vi "Calculate CO2 (2).vi"(7 "Use Channel":u8=1 min=1 max=4, 9 "BreathDuration":dbl, 10 "Daq Needed":T1 {"Current Settings"."Pump" items=["Pump 0", "Pump 1", "Pump 2", "Pump 3", "Pump 4", "Pump 5"]; "Current Settings"."Chart X axis Timescale" min=20 max=180 step=1; "Current Settings"."RunTime Mode Settings"."Exp. Gas Tank" items=["0.07", "0.031", "0.877", "1.863", "3.881", "5.790", "7.688", "6.000"]; "Current Settings"."RunTime Mode Settings"."Insp. Gas Tank" items=["0.07", "0.031", "0.877", "1.863", "3.881", "5.790", "7.688", "6.000"]; "Current Settings"."RunTime Mode Settings"."I:E Ratio" max=30 scale=0.0..7.0; "Current Settings"."RunTime Mode Settings"."Resp Rate Brpm" min=0 max=30 format="%.2f"; "Current Settings"."TE#2 Configuration"."Serial Port"."XOFF Char" format="%.0x"; "Current Settings"."TE#2 Configuration"."Serial Port"."XON Char" format="%.0x"; "Current Settings"."TE#2 Configuration"."Serial Port"."flow control" items=["None"=0, "XON/XOFF"=1, "RTS/CTS"=2, "DTR/DSR"=4]; "Current Settings"."TE#2 Configuration"."Serial Port"."stop bits" items=["1.0"=10, "1.5"=15, "2.0"=20]; "Current Settings"."TE#2 Configuration"."Serial Port"."data bits" min=5 max=8 step=1; "Current Settings"."TE#2 Configuration"."Serial Port"."baud rate" items=["75"=75, "110"=110, "134"=134, "150"=150, "300"=300, "600"=600, "1200"=1200, "1800"=1800, "2400"=2400, "4800"=4800, "7200"=7200, "9600"=9600, "14400"=14400, "19200"=19200, "28800"=28800, "38400"=38400, "56000"=56000, "57600"=57600, "115200"=115200, "128000"=128000, "230400"=230400]; "Current Settings"."TE#2 Configuration"."Serial Port"."termination char" format="%.0x"; "Current Settings"."TE#1 Configuration"."Serial Port"."XOFF Char" format="%.0x"; "Current Settings"."TE#1 Configuration"."Serial Port"."XON Char" format="%.0x"; "Current Settings"."TE#1 Configuration"."Serial Port"."flow control" items=["None"=0, "XON/XOFF"=1, "RTS/CTS"=2, "DTR/DSR"=4]; "Current Settings"."TE#1 Configuration"."Serial Port"."stop bits" items=["1.0"=10, "1.5"=15, "2.0"=20]; "Current Settings"."TE#1 Configuration"."Serial Port"."data bits" min=5 max=8 step=1; "Current Settings"."TE#1 Configuration"."Serial Port"."baud rate" items=["75"=75, "110"=110, "134"=134, "150"=150, "300"=300, "600"=600, "1200"=1200, "1800"=1800, "2400"=2400, "4800"=4800, "7200"=7200, "9600"=9600, "14400"=14400, "19200"=19200, "28800"=28800, "38400"=38400, "56000"=56000, "57600"=57600, "115200"=115200, "128000"=128000, "230400"=230400]; "Current Settings"."TE#1 Configuration"."Serial Port"."termination char" format="%.0x"; "Current Settings"."Capnometer Configuration"."Device" items=["None", "TidalWave", "LoFlow / Canary", "Capnogard"]; "Current Settings"."Capnometer Configuration"."Serial Port"."XOFF Char" format="%.0x"; "Current Settings"."Capnometer Configuration"."Serial Port"."XON Char" format="%.0x"; "Current Settings"."Capnometer Configuration"."Serial Port"."flow control" items=["None"=0, "XON/XOFF"=1, "RTS/CTS"=2, "DTR/DSR"=4]; "Current Settings"."Capnometer Configuration"."Serial Port"."stop bits" items=["1.0"=10, "1.5"=15, "2.0"=20]; "Current Settings"."Capnometer Configuration"."Serial Port"."data bits" min=5 max=8 step=1; "Current Settings"."Capnometer Configuration"."Serial Port"."baud rate" items=["75"=75, "110"=110, "134"=134, "150"=150, "300"=300, "600"=600, "1200"=1200, "1800"=1800, "2400"=2400, "4800"=4800, "7200"=7200, "9600"=9600, "14400"=14400, "19200"=19200, "28800"=28800, "38400"=38400, "56000"=56000, "57600"=57600, "115200"=115200, "128000"=128000, "230400"=230400]; "Current Settings"."Capnometer Configuration"."Serial Port"."termination char" format="%.0x"; "Current Settings"."DAQx Settings"."Analog Output Settings (Volts)" format="%#.3g"; "Current Settings"."DAQx Settings"."Duty Cycle" min=10.0 max=90.0 format="%.1g"; "Current Settings"."DAQx Settings"."Frequency" min=20.0 max=200.0; "Current Settings"."DataLogging Settings"."Data File Duration (Minutes)" min=2 max=200 format="%#.2g"; "Current Settings"."Calibration Settings"."Tolerance #2" min=2 max=4096; "Current Settings"."Calibration Settings"."Cal. Average" min=2 max=4096; "Current Settings"."Test Settings"."Test Sensor ID" items=["(select)", "RB", "YC", "", "Other"]}, 11 "Processed Variables":T9 {"Chamber Temperature" format="%.2f"; "Ambient Temperature" format="%.2f"; "Bath Temperature" format="%.2f"; "Det. Temperature" format="%.2f"; "Detector Chl 4" format="%.2g"; "Detector Chl 3" format="%.2g"; "Ref CO2" format="%.2g"; "Detector Chl 2" format="%.2g"; "Film Temperature" format="%.2f"; "Humidity" format="%.2f"; "Detector Chl 1" format="%.2g"}) -> (1 "RR Out":dbl, 2 "Raws":sgl[](array[numeric]), 3 "ETCO2 Out":dbl, 4 "New Breath Found":bool)   [LabVIEW 2015]
uses:
  Controls/Processed Variables.ctl
  Controls/DAQ Needed.ctl
  Controls/AirPump Controls.ctl
  Controls/IE Ratio knob.ctl
  Controls/UI Settings.ctl
  Controls/Aux CO2 Control.ctl
  Controls/Serial Visa Control.ctl
  Controls/Aux CO2 Selector.ctl
  Controls/Aux TE Control.ctl
  Controls/Queues And Others.ctl
  Miscellaneous/Globals.vi
panel:
  in  "Use New V2C":bool=TRUE
  out "PeakCO2Out":dbl
  # "Note: Setting Brpm to zero will\ndisable Insp / Exp digital output."
  # "mmHg"
  # "pts"
  # "tolerance"
  # "AN5 (Temp 1)"
  # "AN6 (Temp 2)"
  # "AN7 (Temp 3)"
  # "AN8 (T FET)"
  # "AN0 (T POT)"
  # "Tref (Set Pt))"
  # "(Spare)"
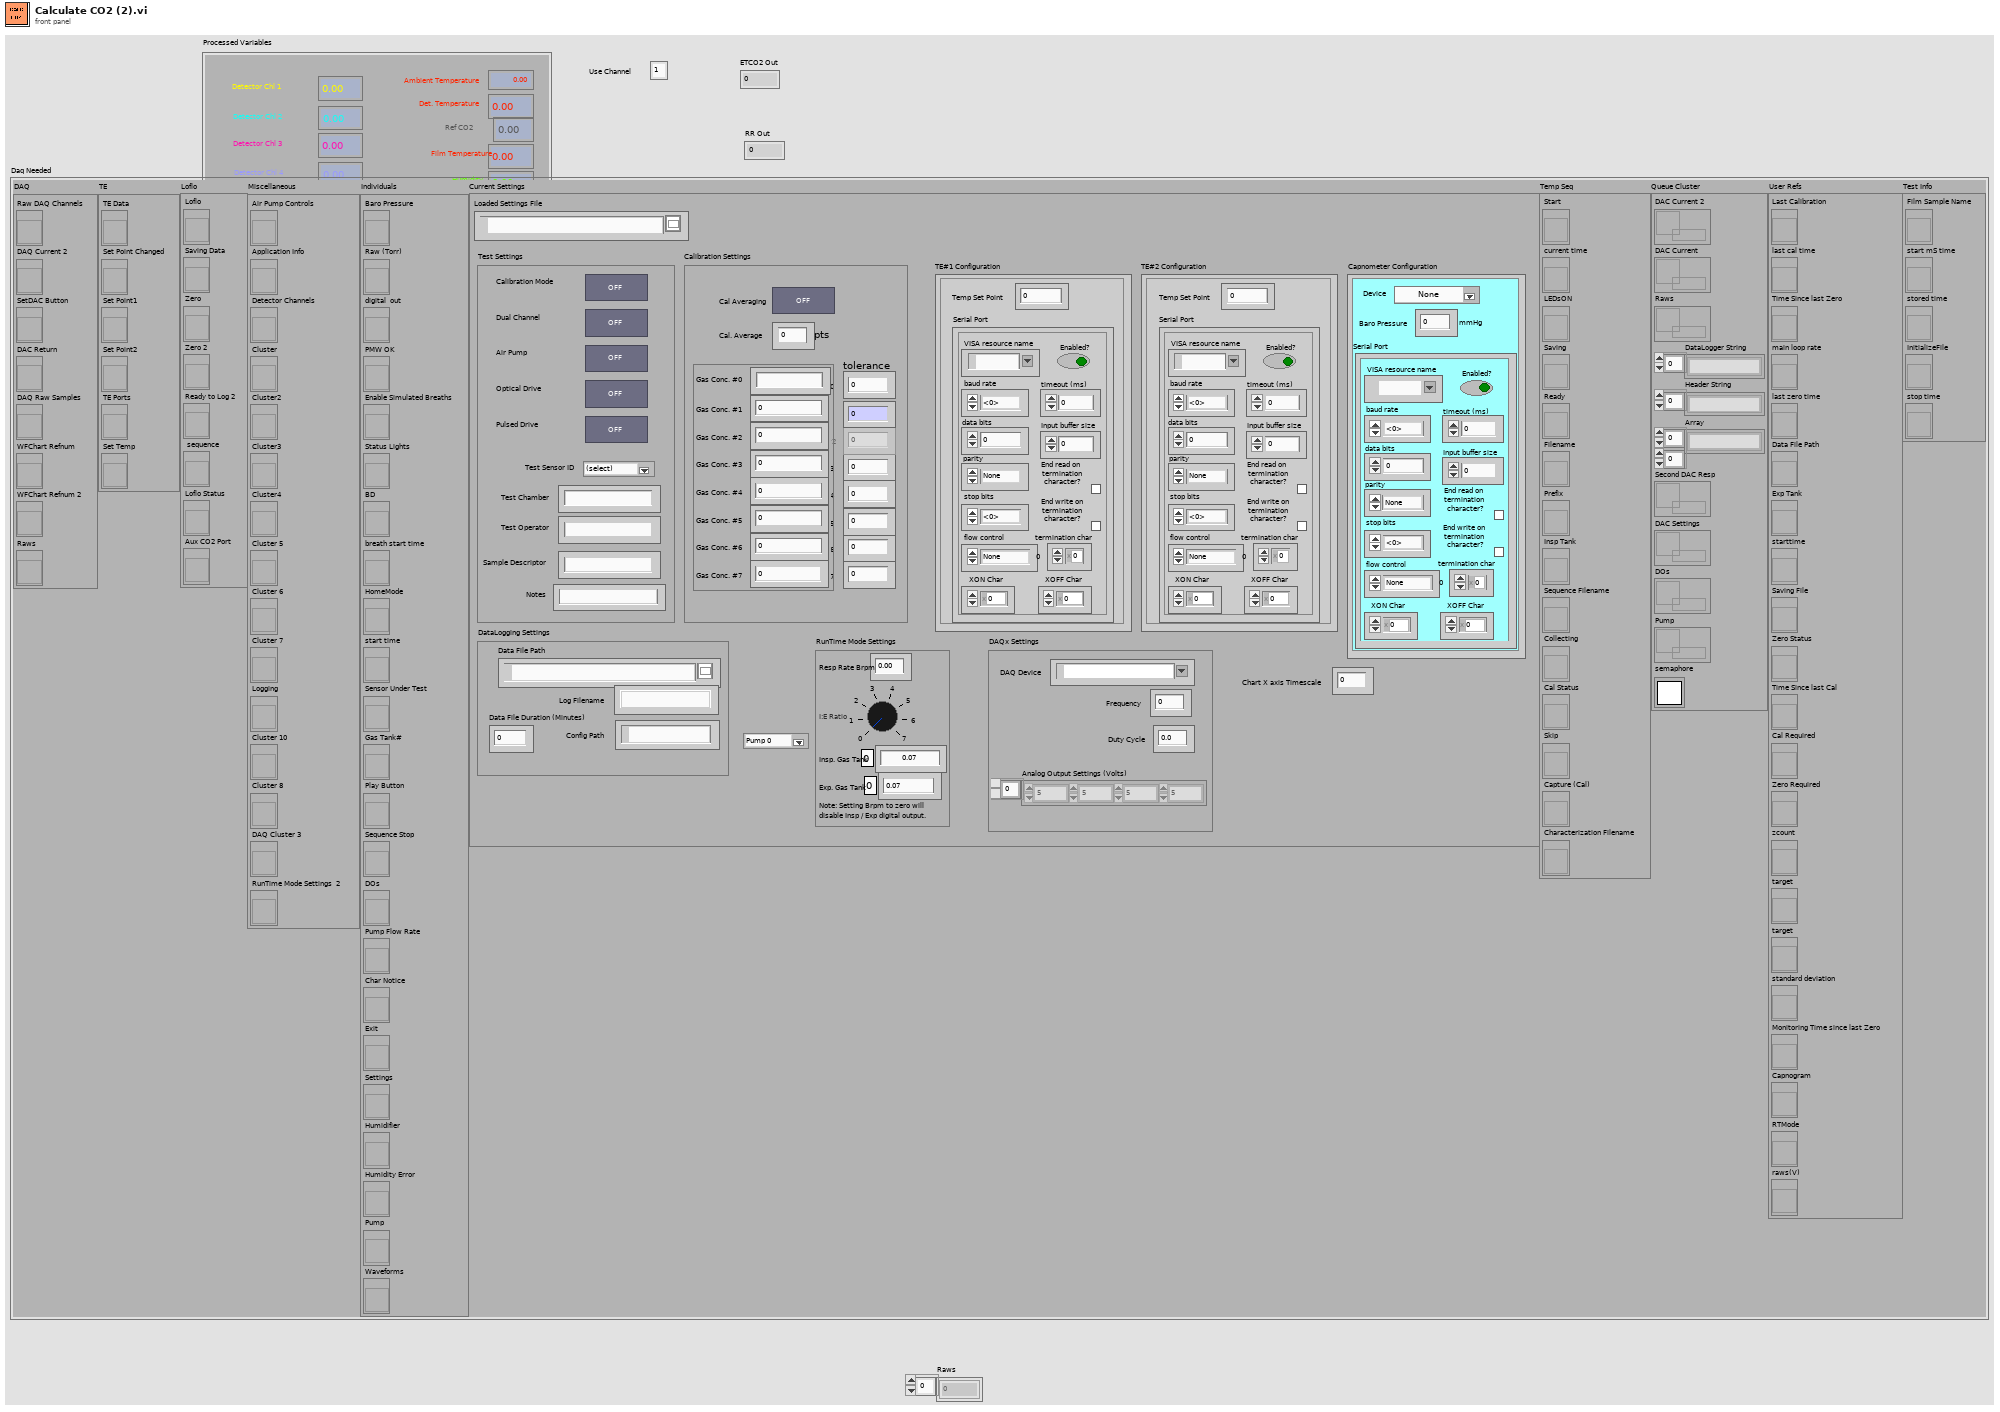
[diagram p1: front panel]
types:
  T1 = typedef "DAQ Needed.ctl" = cluster{"DAQ":cluster{"Raw DAQ Channels":refnum<vi>, "DAQ Current 2":refnum<vi>, "SetDAC Button":refnum<vi>, "DAC Return":refnum<vi>, "DAQ Raw Samples":refnum<vi>, "WFChart Refnum":refnum<vi>, "WFChart Refnum 2":refnum<vi>, "Raws":refnum<vi>}, "TE":cluster{"TE Data":refnum<vi>, "Set Point Changed":refnum<vi>, "Set Point1":refnum<vi>, "Set Point2":refnum<vi>, "TE Ports":refnum<vi>, "Set Temp":refnum<vi>}, "Loflo":cluster{"Loflo":refnum<vi>, "Saving Data":refnum<vi>, "Zero":refnum<vi>, "Zero 2":refnum<vi>, "Ready to Log 2":refnum<vi>, " sequence":refnum<vi>, "Loflo Status ":refnum<vi>, "Aux CO2 Port":refnum<vi>}, "Miscellaneous":cluster{"Air Pump Controls":refnum<vi>, "Application Info":refnum<vi>, "Detector Channels ":refnum<vi>, "Cluster":refnum<vi>, "Cluster2":refnum<vi>, "Cluster3":refnum<vi>, "Cluster4":refnum<vi>, "Cluster 5":refnum<vi>, "Cluster 6":refnum<vi>, "Cluster 7":refnum<vi>, "Logging":refnum<vi>, "Cluster 10":refnum<vi>, "Cluster 8":refnum<vi>, "DAQ Cluster 3":refnum<vi>, "RunTime Mode Settings  2":refnum<vi>}, "Individuals":cluster{"Baro Pressure":refnum<vi>, "Raw (Torr)":refnum<vi>, "digital  out":refnum<vi>, "PMW OK":refnum<vi>, "Enable Simulated Breaths":refnum<vi>, "Status Lights":refnum<vi>, "BD":refnum<vi>, "breath start time":refnum<vi>, "HomeMode":refnum<vi>, "start time":refnum<vi>, "Sensor Under Test":refnum<vi>, "Gas Tank#":refnum<vi>, "Play Button":refnum<vi>, "Sequence Stop":refnum<vi>, "DOs":refnum<vi>, "Pump Flow Rate":refnum<vi>, "Char Notice":refnum<vi>, "Exit":refnum<vi>, "Settings":refnum<vi>, "Humidifier":refnum<vi>, "Humidity Error":refnum<vi>, "Pump":refnum<vi>, "Waveforms":refnum<vi>}, "Current Settings":T2, "Temp Seq":cluster{"Start":refnum<vi>, "current time":refnum<vi>, "LEDsON":refnum<vi>, "Saving":refnum<vi>, "Ready":refnum<vi>, "Filename":refnum<vi>, "Prefix":refnum<vi>, "Insp Tank":refnum<vi>, "Sequence Filename":refnum<vi>, "Collecting":refnum<vi>, "Cal Status":refnum<vi>, "Skip":refnum<vi>, "Capture (Cal)":refnum<vi>, "Characterization Filename":refnum<vi>}, "Queue Cluster":T7, "User Refs":cluster{"Last Calibration":refnum<vi>, "last cal time":refnum<vi>, "Time Since last Zero":refnum<vi>, "main loop rate":refnum<vi>, "last zero time":refnum<vi>, "Data File Path":refnum<vi>, "Exp Tank":refnum<vi>, "starttime":refnum<vi>, "Saving File":refnum<vi>, "Zero Status":refnum<vi>, "Time Since last Cal":refnum<vi>, "Cal Required":refnum<vi>, "Zero Required":refnum<vi>, "zcount":refnum<vi>, "target":refnum<vi>, "target":refnum<vi>, "standard deviation":refnum<vi>, "Monitoring Time since last Zero":refnum<vi>, "Capnogram":refnum<vi>, "RTMode":refnum<vi>, "raws(V)":refnum<vi>}, "Test Info":cluster{"Film Sample Name":refnum<vi>, "start mS time":refnum<vi>, "stored time":refnum<vi>, "InitializeFile":refnum<vi>, "stop time":refnum<vi>}}
  T2 = typedef "UI Settings.ctl" = cluster{"Loaded Settings File":path, "Test Settings":cluster{"Dual Channel":bool, "Air Pump":bool, "Optical Drive":bool, "Pulsed Drive":bool, "Calibration Mode":bool, "Test Sensor ID":u16, "Test Chamber":string, "Test Operator":string, "Sample Descriptor":string, "Notes":string}, "Calibration Settings":cluster{"Cal. Average":u16, "Cal Averaging":bool, "Tolerance #0":sgl, "Tolerance #7":sgl, "Tolerance #6":sgl, "Tolerance #5":sgl, "Tolerance #4":sgl, "Tolerance #3":sgl, "Tolerance #2":sgl, "Tolerance #1":sgl, "Gas Tank Settings":cluster{"Gas Conc. #0":string, "Gas Conc. #1":sgl, "Gas Conc. #2":sgl, "Gas Conc. #3":sgl, "Gas Conc. #4":sgl, "Gas Conc. #5":sgl, "Gas Conc. #6":sgl, "Gas Conc. #7":sgl}}, "DataLogging Settings":cluster{"Data File Path":path, "Data File Duration (Minutes)":sgl, "Log Filename":string, "Config Path":path}, "DAQx Settings":cluster{"DAQ Device":tag, "Frequency":dbl, "Duty Cycle":dbl, "Analog Output Settings (Volts)":sgl[]}, "Capnometer Configuration":T3, "TE#1 Configuration":T6, "TE#2 Configuration":T6, "RunTime Mode Settings ":cluster{"Resp Rate Brpm ":sgl, "I:E Ratio":u8, "Insp. Gas Tank":u16, "Exp. Gas Tank":u16}, "Chart X axis Timescale":u16, "Pump":u16}
  T3 = typedef "Aux CO2 Control.ctl" = cluster{"Serial Port":T4, "Baro Pressure":u32, "Device":T5}
  T4 = typedef "Serial Visa Control.ctl" = cluster{"termination char":u8, "End read on termination character?":bool, "Enabled?":bool, "VISA resource name":refnum<visa-resource-name>, "baud rate":u32, "data bits":u16, "parity":enum16{"None", "Odd", "Even", "Mark", "Space"}, "stop bits":u16, "flow control":u16, "timeout (ms)":u32, "Input buffer size":u32, "End write on termination character?":bool, "XON Char":u8, "XOFF Char":u8}
  T5 = typedef "Aux CO2 Selector.ctl" = u16
  T6 = typedef "Aux TE Control.ctl" = cluster{"Temp Set Point":sgl, "Serial Port":T4}
  T7 = typedef "Queues And Others.ctl" = cluster{"DAC Current 2":refnum<queue>, "DAC Current":refnum<queue>, "Raws":refnum<queue>, "DataLogger String":string[], "Header String":string[], "Array":string[][], "Second DAC Resp":refnum<queue>, "DAC Settings":refnum<queue>, "DOs":refnum<queue>, "Pump":refnum<queue>, "semaphore":T8}
  T8 = typedef "Semaphore RefNum" = refnum<k1>
  T9 = typedef "Processed Variables.ctl" = cluster{"Detector Chl 1":sgl, "Humidity":dbl, "Film Temperature":dbl, "Detector Chl 2":sgl, "Ref CO2":sgl, "Detector Chl 3":sgl, "Detector Chl 4":sgl, "Det. Temperature":dbl, "Bath Temperature":dbl, "Ambient Temperature":dbl, "rt Baro Pressure":u16, "Chamber Temperature":dbl}
  T10 = typedef "Calibration Coefficients.ctl" = cluster{"CalFile Used":path, "TYPE":string, "DATE":string, "Humidity":sgl, "Chamber Temp":dbl, "CO2_calgas":dbl, "V_(RA,5mA)":dbl, "V_(RA,15mA)":dbl, "mI":dbl, "V_0d_ImA (actual)":dbl, "V_6d_ImA (actual)":dbl, "I_span":dbl, "DAC":u16, "A":dbl, "B":dbl, "C":dbl, "D":dbl, "V6d":dbl, "A'":dbl, "B'":dbl, "C'":dbl, "D'":dbl, "V0d":dbl, "CalDate":string, "CalTime":string, "duration":dbl, "Detector Channel":string, "a2":dbl, "a3":dbl, "a4":dbl, "a5":dbl, "b2":dbl, "c2":dbl, "b3":dbl, "c3":dbl, "b4":dbl, "c4":dbl, "b5":dbl, "c5":dbl, "a7":dbl, "a8":dbl, "a9":dbl, "a10":dbl, "b7":dbl, "b8":dbl, "b9":dbl, "b10":dbl, "c7":dbl, "c8":dbl, "c9":dbl, "c10":dbl, "cal_offs_adj":dbl, "cal_gain_adj":dbl, "C6d":dbl, "C0d":dbl, "Cal_currernt":dbl, "C2V":u16, "V2C":u16, "Zero Date":string, "Zero Time":string, "Number of Zeroes":u16, "V_(()d, average)":dbl, "V_offs ":dbl, "G_adj":dbl, "Pump Flow Rate":u16, "Zero Required? ":bool, "Calibrate Required?":bool, "cal_utc":dbl, "zero_utc":dbl, "Elapsed Time":dbl, "PCB":string, "m0":dbl, "b0":dbl}
  T11 = typedef "IE Ratio knob.ctl" = u8
  T12 = cluster{"pk":sgl, "RawCO2":sgl, "Uncal'd":sgl, "Avg_Hum":sgl, "Avg'd CO2":sgl, "Home_CO2":sgl, "Home_Ref":sgl, "Home_Hum":sgl, " Home Temp":dbl, "Pump Flow Rate":u16, "I:E Ratio":T11, "Brpm":sgl, "Sim Breaths":bool, "GasTank":u8}
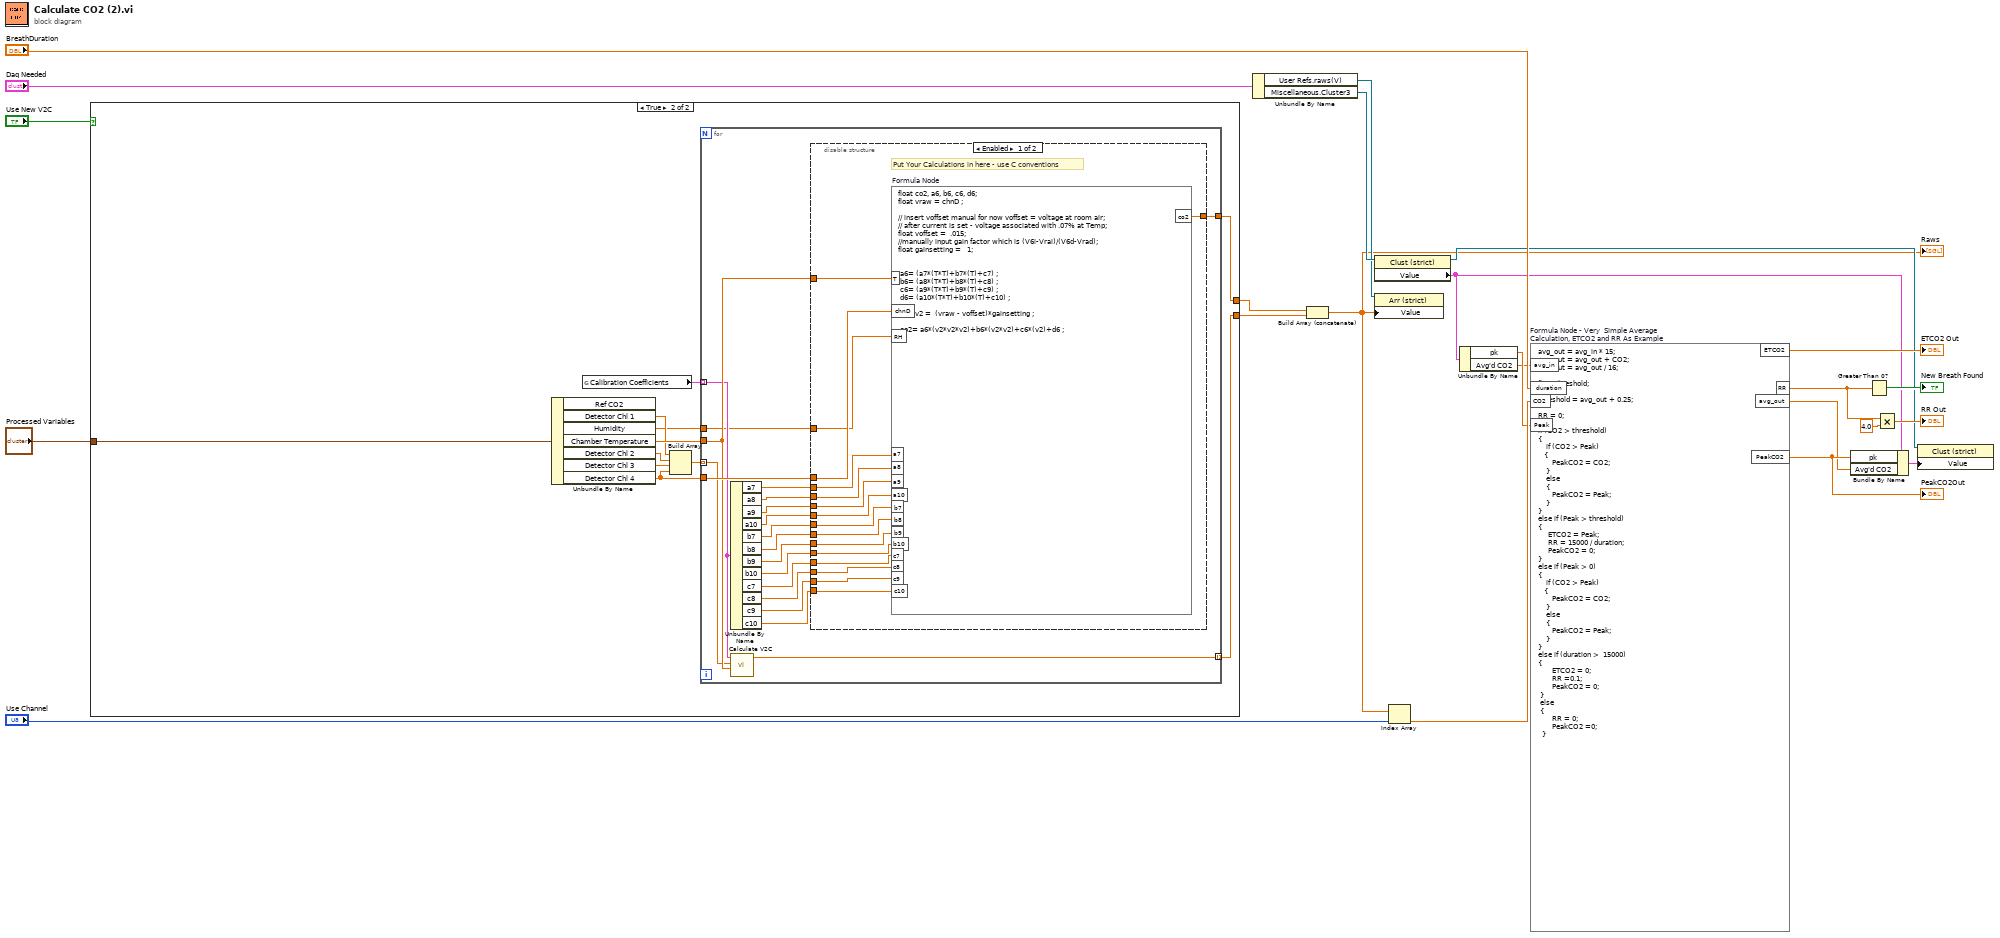
[diagram p0: block diagram]
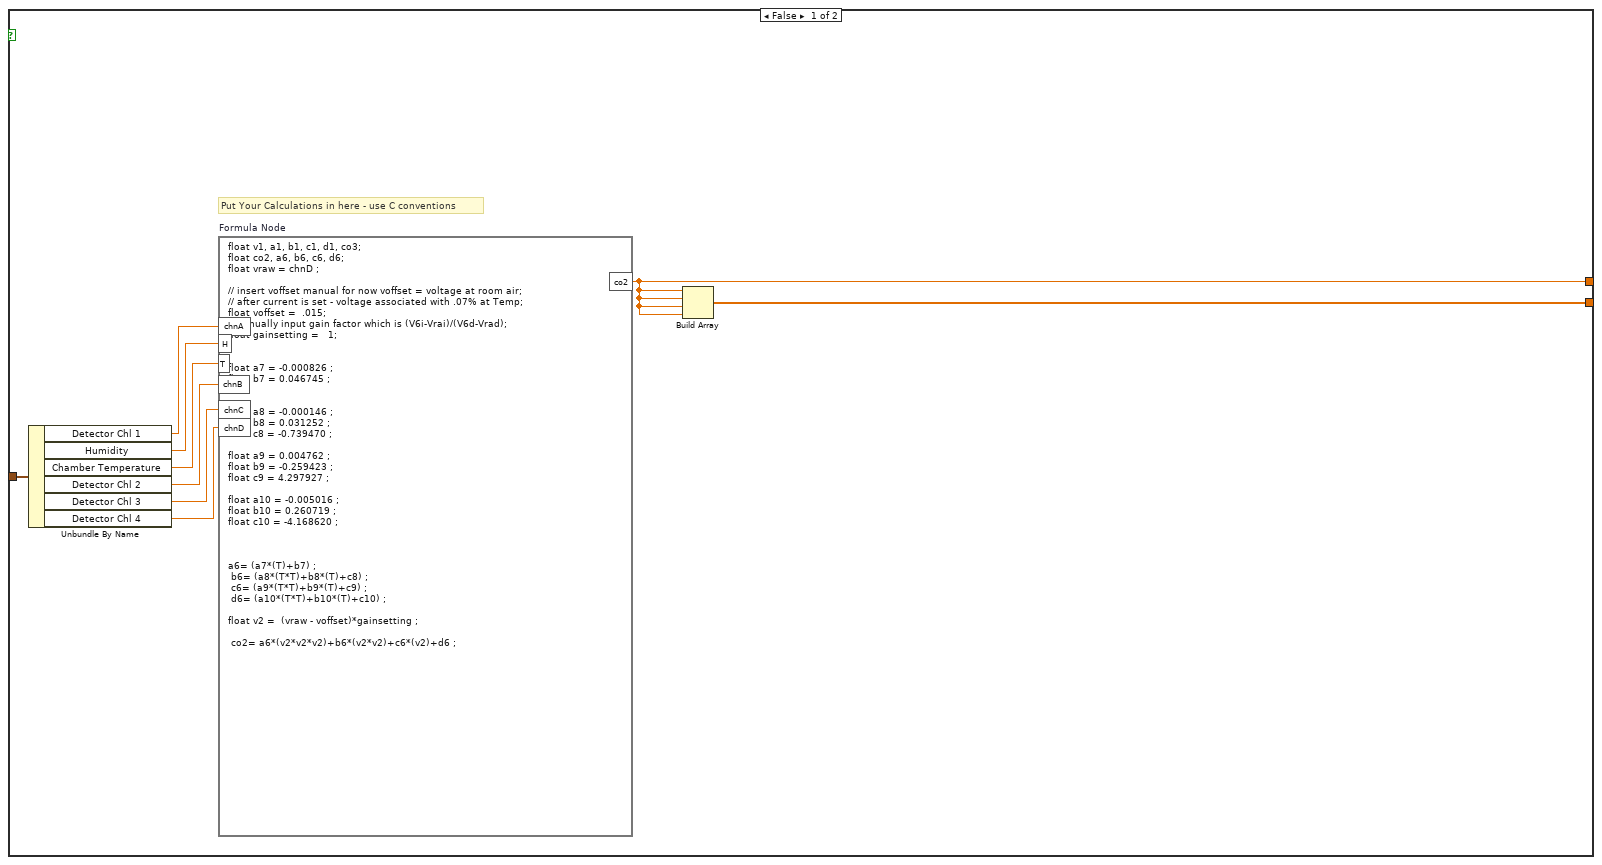
[diagram p2: hidden frame]
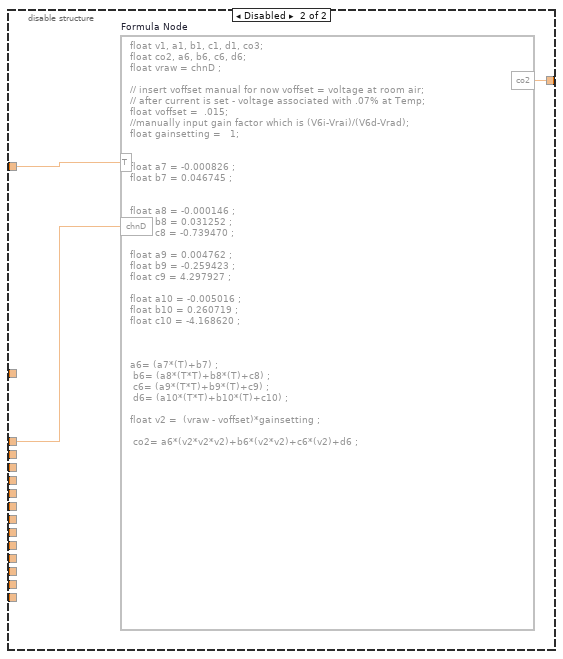
[diagram p3: hidden frame]
diagram:
  n1 = case shown="True" "Use New V2C" {
    tunnel: "Processed Variables" -> [w26 w43]
    tunnel: [w25 w41] -> w12
    tunnel: [w24 w35] -> w13
    frame False {
      # "Put Your Calculations in here - use C conventions"
      n2 = Unbundle By Name(w26) -> ("Detector Chl 1"=w32:sgl, "Humidity"=w29:dbl, "Chamber Temperature"=w30:dbl, "Detector Chl 2"=w28:sgl, "Detector Chl 3"=w27:sgl, "Detector Chl 4"=w31:sgl)
      n3 = formula code="float\tv1, a1, b1, c1, d1, co3;\t\t\nfloat\tco2, a6, b6, c6, d6;\t\t\nfloat\tvraw =\tchnD\t;\n\t\t\t\n// insert voffset manual for now voffset = voltage at room air;\t\t\t\n// after current is set - voltage associated with .07% at Temp;\t\t\t\nfloat\tvoffset =\t\t.015;\n//manually input gain factor which is (V6i-Vrai)/(V6d-Vrad);\t\t\t\nfloat\tgainsetting = \t\t1;\n\t\t\t\n\t\t\t\nfloat\ta7 =\t-0.000826\t;\nfloat\tb7 =\t0.046745\t;\n\t\t\t\n\t\t\t\nfloat\ta8 =\t-0.000146\t;\nfloat\tb8 =\t0.031252\t;\nfloat\tc8 =\t-0.739470\t;\n\t\t\t\nfloat\ta9 =\t0.004762\t;\nfloat\tb9 =\t-0.259423\t;\nfloat\tc9 =\t4.297927\t;\n\t\t\t\nfloat\ta10 =\t-0.005016\t;\nfloat\tb10 =\t0.260719\t;\nfloat\tc10 =\t-4.168620\t;\n\t\t\t\n\n\t\t\t\na6=\t(a7*(T)+b7)\t;\n\tb6=\t(a8*(T*T)+b8*(T)+c8)\t;\n\tc6=\t(a9*(T*T)+b9*(T)+c9)\t;\n\td6=\t(a10*(T*T)+b10*(T)+c10)\t;\n\t\t\t\nfloat\tv2 = \t(vraw - voffset)*gainsetting\t;\n\t\t\t\n\tco2=\ta6*(v2*v2*v2)+b6*(v2*v2)+c6*(v2)+d6\t;"("chnA"=w32, "chnD"=w31, "T"=w30, "H"=w29, "chnB"=w28, "chnC"=w27) -> ("co2"=w24:dbl)
      n4 = Build Array(w24, w24, w24, w24) -> (w25:dbl[])
    }
    frame True {
      n5 = Unbundle By Name(w43) -> ("Detector Chl 1"=w36:sgl, "Humidity"=w34:dbl, "Chamber Temperature"=w42:dbl, "Detector Chl 2"=w37:sgl, "Detector Chl 3"=w38:sgl, "Detector Chl 4"=w39:sgl)  [unwired: 1 out]
      n6 = global read "Globals.vi" "Calibration Coefficients"() -> (w33:T10[])
      n7 = Build Array(w36, w37, w38, w39) -> (w40:sgl[])
      n8 = for {
        tunnel: w33 -> [w48] mode=indexing
        tunnel: w39 -> [w50]
        tunnel: w42 -> [w49]
        tunnel: [w47] -> w41 mode=indexing
        tunnel: [w46] -> w35
        tunnel: w40 -> [w45] mode=indexing
        tunnel: w34 -> [w44]
        n9 = Unbundle By Name(w48) -> ("a7"=w51:dbl, "a8"=w52:dbl, "a9"=w53:dbl, "a10"=w54:dbl, "b7"=w55:dbl, "b8"=w56:dbl, "b9"=w57:dbl, "b10"=w58:dbl, "c7"=w59:dbl, "c8"=w60:dbl, "c9"=w61:dbl, "c10"=w62:dbl)
        n10 = call "Calculate V2C.vi"("Tcal_Chamber"=w49, "Voltage In"=w45, "Calibration Coefficients"=w48) -> ("CO2 Out"=w47:dbl)  [unwired: 4 in, 4 out]
        n11 = disable-structure shown="Enabled" {
          disable-tunnel: w50 -> [w78 w81]
          disable-tunnel: w49 -> [w77 w80]
          disable-tunnel: [w76 w79] -> w46
          disable-tunnel: w62 -> [w75 _]
          disable-tunnel: w61 -> [w74 _]
          disable-tunnel: w60 -> [w73 _]
          disable-tunnel: w59 -> [w72 _]
          disable-tunnel: w58 -> [w71 _]
          disable-tunnel: w57 -> [w70 _]
          disable-tunnel: w56 -> [w69 _]
          disable-tunnel: w55 -> [w68 _]
          disable-tunnel: w54 -> [w67 _]
          disable-tunnel: w53 -> [w66 _]
          disable-tunnel: w52 -> [w65 _]
          disable-tunnel: w51 -> [w64 _]
          disable-tunnel: w44 -> [w63 _]
          frame Enabled {
            # "Put Your Calculations in here - use C conventions"
            n12 = formula code="float\tco2, a6, b6, c6, d6;\t\t\nfloat\tvraw =\tchnD\t;\n\t\t\t\n// insert voffset manual for now voffset = voltage at room air;\t\t\t\n// after current is set - voltage associated with .07% at Temp;\t\t\t\nfloat\tvoffset =\t\t.015;\n//manually input gain factor which is (V6i-Vrai)/(V6d-Vrad);\t\t\t\nfloat\tgainsetting = \t\t1;\n\n\n\ta6=\t(a7*(T*T)+b7*(T)+c7)\t;\n\tb6=\t(a8*(T*T)+b8*(T)+c8)\t;\n\tc6=\t(a9*(T*T)+b9*(T)+c9)\t;\n\td6=\t(a10*(T*T)+b10*(T)+c10)\t;\n\t\t\t\nfloat\tv2 = \t(vraw - voffset)*gainsetting\t;\n\t\t\t\n\tco2=\ta6*(v2*v2*v2)+b6*(v2*v2)+c6*(v2)+d6\t;"("chnD"=w78, "T"=w77, "a7"=w64, "a8"=w65, "a9"=w66, "a10"=w67, "b7"=w68, "b8"=w69, "b9"=w70, "b10"=w71, "c7"=w72, "c8"=w73, "c9"=w74, "c10"=w75, "RH"=w63) -> ("co2"=w76:dbl)
          }
          frame Disabled {
            n13 = formula code="float\tv1, a1, b1, c1, d1, co3;\t\t\nfloat\tco2, a6, b6, c6, d6;\t\t\nfloat\tvraw =\tchnD\t;\n\t\t\t\n// insert voffset manual for now voffset = voltage at room air;\t\t\t\n// after current is set - voltage associated with .07% at Temp;\t\t\t\nfloat\tvoffset =\t\t.015;\n//manually input gain factor which is (V6i-Vrai)/(V6d-Vrad);\t\t\t\nfloat\tgainsetting = \t\t1;\n\t\t\t\n\t\t\t\nfloat\ta7 =\t-0.000826\t;\nfloat\tb7 =\t0.046745\t;\n\t\t\t\n\t\t\t\nfloat\ta8 =\t-0.000146\t;\nfloat\tb8 =\t0.031252\t;\nfloat\tc8 =\t-0.739470\t;\n\t\t\t\nfloat\ta9 =\t0.004762\t;\nfloat\tb9 =\t-0.259423\t;\nfloat\tc9 =\t4.297927\t;\n\t\t\t\nfloat\ta10 =\t-0.005016\t;\nfloat\tb10 =\t0.260719\t;\nfloat\tc10 =\t-4.168620\t;\n\t\t\t\n\n\t\t\t\na6=\t(a7*(T)+b7)\t;\n\tb6=\t(a8*(T*T)+b8*(T)+c8)\t;\n\tc6=\t(a9*(T*T)+b9*(T)+c9)\t;\n\td6=\t(a10*(T*T)+b10*(T)+c10)\t;\n\t\t\t\nfloat\tv2 = \t(vraw - voffset)*gainsetting\t;\n\t\t\t\n\tco2=\ta6*(v2*v2*v2)+b6*(v2*v2)+c6*(v2)+d6\t;"("chnD"=w81, "T"=w80) -> ("co2"=w79:dbl)
          }
        }
      }
    }
  }
  n14 = Unbundle By Name("Daq Needed") -> ("User Refs.raws(V)"=w2:refnum<vi>, "Miscellaneous.Cluster3"=w10:refnum<vi>)
  n15 = Build Array (concatenate)(w13, w12) -> (w1:dbl[])
  "Raws" <- w1
  n16 = property class="Clust (strict)"(reference=w10) -> (reference out=w8:refnum<vi>, "Value"=w7:T12)  [unwired: 1 in, 1 out]
  n17 = property class="Arr (strict)"(reference=w2, "Value"=w1) -> ()  [unwired: 1 in, 2 out]
  n18 = Index Array(array=w1, index="Use Channel") -> (element=w14:dbl)
  n19 = Unbundle By Name(w7) -> ("pk"=w9:sgl, "Avg'd CO2"=w4:sgl)
  n20 = formula code="avg_out = avg_in * 15;\navg_out = avg_out + CO2;\navg_out = avg_out / 16;\n\nfloat threshold;\n\nthreshold = avg_out + 0.25;\n\nRR = 0;\n\nif (CO2 > threshold) \n{\n    if (CO2 > Peak)\n   {\n       PeakCO2 = CO2;\n    }\n    else\n    {\n       PeakCO2 = Peak;\n    }\n}\nelse if (Peak > threshold)\n{\n     ETCO2 = Peak;\n     RR = 15000 / duration;  \n     PeakCO2 = 0;\n}\nelse if (Peak > 0)\n{\n    if (CO2 > Peak)\n   {\n       PeakCO2 = CO2;\n    }\n    else\n    {\n       PeakCO2 = Peak;\n    }\n}\nelse if (duration >  15000)\n{\n       ETCO2 = 0;\n       RR =0.1;\n       PeakCO2 = 0;\n }\n else\n {\n       RR = 0;\n       PeakCO2 =0;\n  }" "Formula Node - Very  Simple Average Calculation, ETCO2 and RR As Example"("CO2"=w14, "avg_in"=w4, "duration"="BreathDuration", "Peak"=w9) -> ("avg_out"=w3:dbl, "ETCO2"=→"ETCO2 Out":dbl, "RR"=w19:dbl, "PeakCO2"=w5:dbl)
  "PeakCO2Out" <- w5
  n21 = Bundle By Name(cluster=w7, "pk"=w5, "Avg'd CO2"=w3) -> (w6:T12)
  n22 = Greater Than 0?(x=w19) -> (x > 0?=→"New Breath Found":bool)
  n23 = Multiply(x=w19, y=4.0) -> (x*y=→"RR Out":dbl)
  n24 = property class="Clust (strict)"(reference=w8, "Value"=w6) -> ()  [unwired: 1 in, 2 out]
